vi "Get PCL Decimation.vi"(8 "Error In":errorcluster, 11 "Instrument Addon Refnum In":T1 format="%.0x") -> (0 "Error Out":errorcluster, 2 "PCL Decimation":u32, 3 "Instrument Addon Refnum Out":T1=18446744073709551615 format="%.0x")   [LabVIEW 2018, in "Instrument Addon Scripting API.lvlib"]
doc: "Returns the PCL Decimation value set for the Instrument Addon Custom Device\n\nInput:\nInstrument Addon Refnum In: represents the refference number to an Instrument Addon Custom Device\n\nOutput:\nInstrument Addon Refnum Out: represents the refference number to the Instrument Addon Custom Device provided as an input\nPCL Decimation: represents the PCL Decimation Value of the Instrument Addon Custom Device"
uses:
  Instrument Addon Scripting API.lvlib
  <vilib>/NI Veristand/Custom Device API/Custom Device Item Ref.ctl
  Addon/Addon Shared/SubVIs/Constants.vi
  <vilib>/NI/NI VeriStand Advanced SysDef API/_SubVIs/SysDef.Property.Get.U32.vi
  Addon/Addon Shared/Instrument Addon Shared.lvlib
  <vilib>/NI/NI VeriStand Advanced SysDef API/SysDef API/Advanced System Definition.lvlib
  <vilib>/NI Veristand/Custom Device API/Custom Device API.lvlib
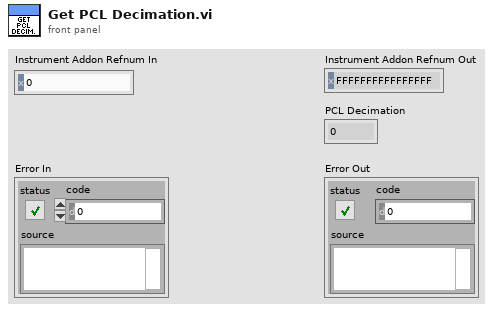
[diagram p1: front panel]
types:
  T1 = typedef "Custom Device API.lvlib/Custom Device Item Ref.ctl" = u64
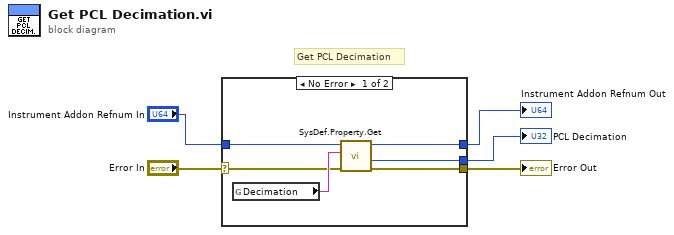
[diagram p0: block diagram]
diagram:
  # "Get PCL Decimation"
  n1 = case shown="No Error" "Error In" {
    selector: "Error In" -> [w10 w13]
    tunnel: "Instrument Addon Refnum In" -> [w7 w12]
    tunnel: [w9 _] -> w4
    tunnel: [w8 w13] -> w3
    tunnel: [w6 w12] -> w1
    frame No Error {
      n2 = global read "Constants.vi" "Decimation"() -> (w11:string)
      n3 = call-poly <vilib>:"SysDef.Property.Get.vi"("error in (no error)"=w10, "Property Name"=w11, "nodeID"=w7) -> ("error out"=w8:errorcluster, "Value out"=w9:u32, "nodeID out"=w6:u64)  [unwired: 5 in, 1 out]
    }
    frame Error {
    }
  }
  "PCL Decimation" <- w4
  "Error Out" <- w3
  "Instrument Addon Refnum Out" <- w1
